vi "RS485_Data_Ctrl.vi"() -> ()   [LabVIEW 2016]
uses:
  <vilib>/Analysis/NI_AALBase.lvlib
  <vilib>/Instr/_visa.llb/VISA Set IO Buffer Mask.ctl
  <vilib>/Instr/_visa.llb/VISA Flush IO Buffer Mask.ctl
  <vilib>/ptbypt/NI_PtbyPt.lvlib
  GEN_2.lvlib
  GEN2_Stat_Addr.ctl
  GEN2_Config_Addr.ctl
  <vilib>/Analysis/1siggen.llb/Ramp Pattern by Samples.vi
  <vilib>/Analysis/3filter.llb/Filter Passband Type.ctl
  <vilib>/Analysis/3filter.llb/Zero Phase Filter (DBL).vi
  <vilib>/Instr/_visa.llb/VISA Configure Serial Port (Instr).vi
  <vilib>/Analysis/1siggen.llb/Ramp Pattern by Delta.vi
  <vilib>/event_ctls.llb/eventvkey.ctl
panel:
  out "Error":cluster{dbl, dbl, dbl[]}[](graph)=[{0.0, 0.005, array[4200 elements]}, {0.0, 0.005, array[4200 elements]}]
  out "Current (Iq)":cluster{dbl, dbl, dbl[]}[](graph)=[{0.0, 0.005, array[4200 elements]}, {0.0, 0.005, array[4200 elements]}]
  out "Iq":dbl=-0.4256019592285156
  in  "which_goal":bool[](array[boolean])=[FALSE, TRUE, TRUE, TRUE]
  in  "ESTOP":bool
  in  "Write Configs":bool
  out "Theta_dot":cluster{"Mean":dbl, "Std":dbl}={"Mean"=0.00022035774236428551, "Std"=0.024452840778427565} {"Std" format="%.4f"; "Mean" format="%.4f"}
  out "Theta_LP":cluster{"Mean":dbl, "Std":dbl}={"Mean"=-0.566546102927532, "Std"=2.22577060098394e-05} {"Std" format="%.4f"; "Mean" format="%.4f"}
  out "Id":cluster{"Mean":dbl, "Std":dbl}={"Mean"=-0.00010110904884186311, "Std"=0.00796473691732965} {"Std" format="%.4f"; "Mean" format="%.4f"}
  in  "MT":cluster{"Expected":sgl, "Tolerance":sgl}
  in  "Find MT":bool
  out "Errors":bool[](array[boolean])=[FALSE, FALSE, FALSE, FALSE, FALSE, FALSE, FALSE, TRUE]
  in  "All config":cluster{"Config Address":T1, dbl}[](array[cluster])=[{"Config Address"=0, 1.0}, {"Config Address"=1, 3.0}, {"Config Address"=2, 8000000.0}, {"Config Address"=3, -0.496978759765625}, {"Config Address"=4, 0.018400000408291817}, {"Config Address"=5, 0.006500000134110451}, {"Config Address"=6, 0.0}, {"Config Address"=7, 0.018400000408291817}, {"Config Address"=8, 0.006500000134110451}, {"Config Address"=9, 0.0}, {"Config Address"=10, 5.0}, {"Config Address"=11, 0.029999999329447746}, {"Config Address"=12, 0.0}, {"Config Address"=13, 10.0}, {"Config Address"=14, 0.0}, {"Config Address"=15, 0.0}, {"Config Address"=16, 100.0}, {"Config Address"=17, 0.0}, {"Config Address"=18, 1.0}, {"Config Address"=19, 5.0}, {"Config Address"=20, 10.0}, {"Config Address"=21, 10.0}, {"Config Address"=22, -3.0}, {"Config Address"=23, 3.0}, {"Config Address"=24, 6.0}, {"Config Address"=25, 60.0}, {"Config Address"=26, 0.0}, {"Config Address"=27, 80.0}, {"Config Address"=28, 100.0}] {"Config Address" items=["ID", "Mode", "Baudrate", "Homing Offset", "Id P gain", "Id I gain", "Id D gain", "Iq P gain", "Iq I gain", "Iq D gain", "Velo P gain", "Velo I gain", "Velo D gain", "Posi P gain", "Posi I gain", "Posi D gain", "DirectForce P", "DirectForce I", "DirectForce D", "Limit Acc Max", "Limit Iq Max", "Limit Velo Max", "Limit Posi Min", "Limit Posi Max", "Voltage Min", "Voltage Max", "Watchdog", "Temperature Low", "Temperature High"]}
  in  "SAVE":bool
  in  "Down_Key":bool
  in  "UP_Key":bool
  out "VKey":T2
  out "Vbus":dbl(graph)=11.93691349029541
  out "Error count":u64=1
  in  "Read Configs":bool
  out "Temperature":cluster{dbl, dbl, dbl}(graph)={27.25, 43.0078125, 41.5625}
  out "Iq":cluster{dbl, dbl}(graph)={-0.4256019592285156, -0.43746575713157654}
  out "Id":cluster{dbl, dbl}(graph)={0.0019982189405709505, 0.0}
  out "Theta":cluster{dbl, dbl}(graph)={-0.5665233731269836, -0.5707402229309082}
  out "Theta_dot":cluster{dbl, dbl}(graph)={-0.004696944262832403, 0.012627856805920601}
  in  "ID":u8=1
  in  "Read":bool=TRUE
  in  "PID0":bool
  in  "P0.001":bool
  in  "D0.5":bool
  in  "P0.0002":bool
  in  "send sine":bool
  in  "2state":bool
  in  "Chirp":i32(listbox)=3
  out "Waveform Graph":cluster{dbl, dbl, dbl[]}(graph)={0.0, 0.005, array[4200 elements]}
  in  "Sample_rate":dbl=200.0 format="%#_13g"
  out "Theta_LP":dbl=-0.5665233731269836
  in  "send chirp":bool
  in  "Enable":bool
  in  "DISABLE":bool
  in  "Write_Mode":bool
  in  "Mode":i32(listbox)=3
  in  "Write_Limits":bool
  in  "Limits":cluster{"Iq&Id":sgl, "Velo":sgl, "Acc":sgl}={"Iq&Id"=10.0, "Velo"=10.0, "Acc"=5.0}
  in  "Goal":T3
  in  "PID_F":cluster{"P":sgl, "I":sgl, "D":sgl}={"P"=100.0, "I"=0.0, "D"=1.0}
  in  "PID_P":cluster{"P":sgl, "I":sgl, "D":sgl}={"P"=10.0, "I"=0.0, "D"=0.0}
  out "Iq":cluster{"Mean":dbl, "Std":dbl}={"Mean"=-0.4106114786118269, "Std"=0.012899504647628292} {"Std" format="%.4f"; "Mean" format="%.4f"}
  in  "amplitude":dbl=2.0 format="%#_13g"
  in  "Time":dbl=20.0 format="%#_13g"
  in  "frq_2":dbl=0.2 format="%#_13g"
  in  "frq_1":dbl format="%#_13g"
  in  "stop":bool
  in  "Write_Goal":bool
  in  "PID_IqId":cluster{"P":sgl, "I":sgl, "D":sgl}={"P"=0.0184, "I"=0.0065, "D"=0.0}
  in  "PID_V":cluster{"P":sgl, "I":sgl, "D":sgl}={"P"=5.0, "I"=0.03, "D"=0.0}
  in  "Write_PID":bool
  in  "Baudrate":u32=8000000
  in  "Buffer Size":u32=150000
  in  "COM":refnum<visa-resource-name>="COM13"
  # "0: WARN COMM\n1: WARN OVTEMP\n2: ERR ABS POSI\n3: ERR WTCHDOG\n4: ERR JOINT LMT\n5: ERR HW FAULT\n6: ERR INIT"
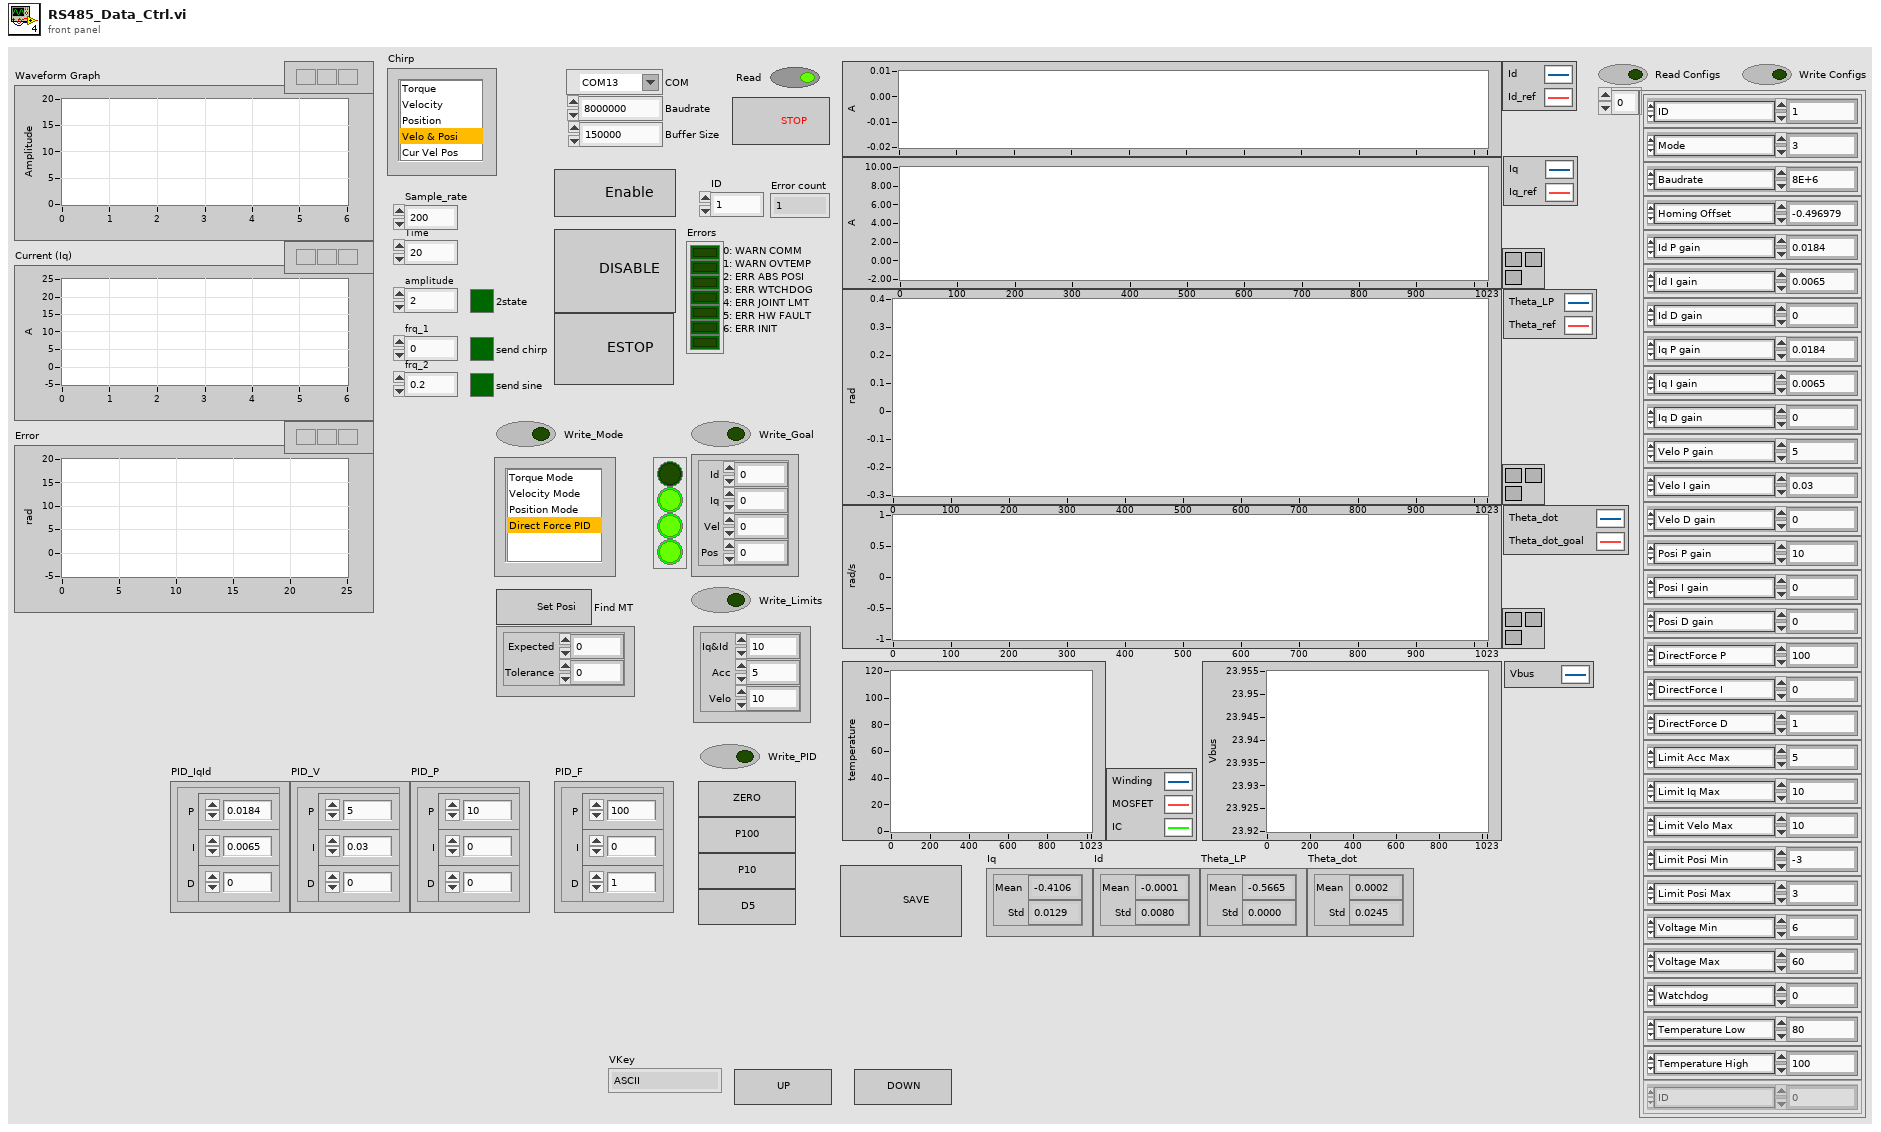
[diagram p1: front panel]
types:
  T1 = typedef "GEN_2.lvlib/GEN2_Config_Addr.ctl" = u8
  T2 = typedef "eventvkey.ctl" = enum16{"ASCII", "Enter", "Return", "Shift", "Ctrl", "Alt", "Cmd", "Opt", "Caps", "NumLock", "Clear", "Break", "Up", "Down", "Left", "Right", "Insert", "Delete", "Home", "End", "PageUp", "PageDown", "Escape", "Help", "Pause", "ScrollLock", "F1", "F2", "F3", "F4", "F5", "F6", "F7", "F8", "F9", "F10", "F11", "F12", "F13", "F14", "F15", "F16", "F17", "F18", "F19", "F20", "F21", "F22", "F23", "F24", "Play", "VolumeUp", "VolumeDown", "Mute", "Two Byte Char"}
  T3 = cluster{"Id":sgl, "Iq":sgl, "Pos":sgl, "Vel":sgl}
  T4 = typedef "NI_AALBase.lvlib/Filter Passband Type.ctl" = enum32{"Lowpass", "Highpass", "Bandpass", "Bandstop"}
  T5 = typedef "VISA Flush IO Buffer Mask.ctl" = u16
  T6 = typedef "VISA Set IO Buffer Mask.ctl" = u16
  T7 = typedef "GEN_2.lvlib/GEN2_Stat_Addr.ctl" = u8
  T8 = cluster{"filter structure":enum32{"IIR 2nd Order", "IIR 4th Order"}, "Reverse Coefficients":dbl[], "Forward Coefficients":dbl[]}
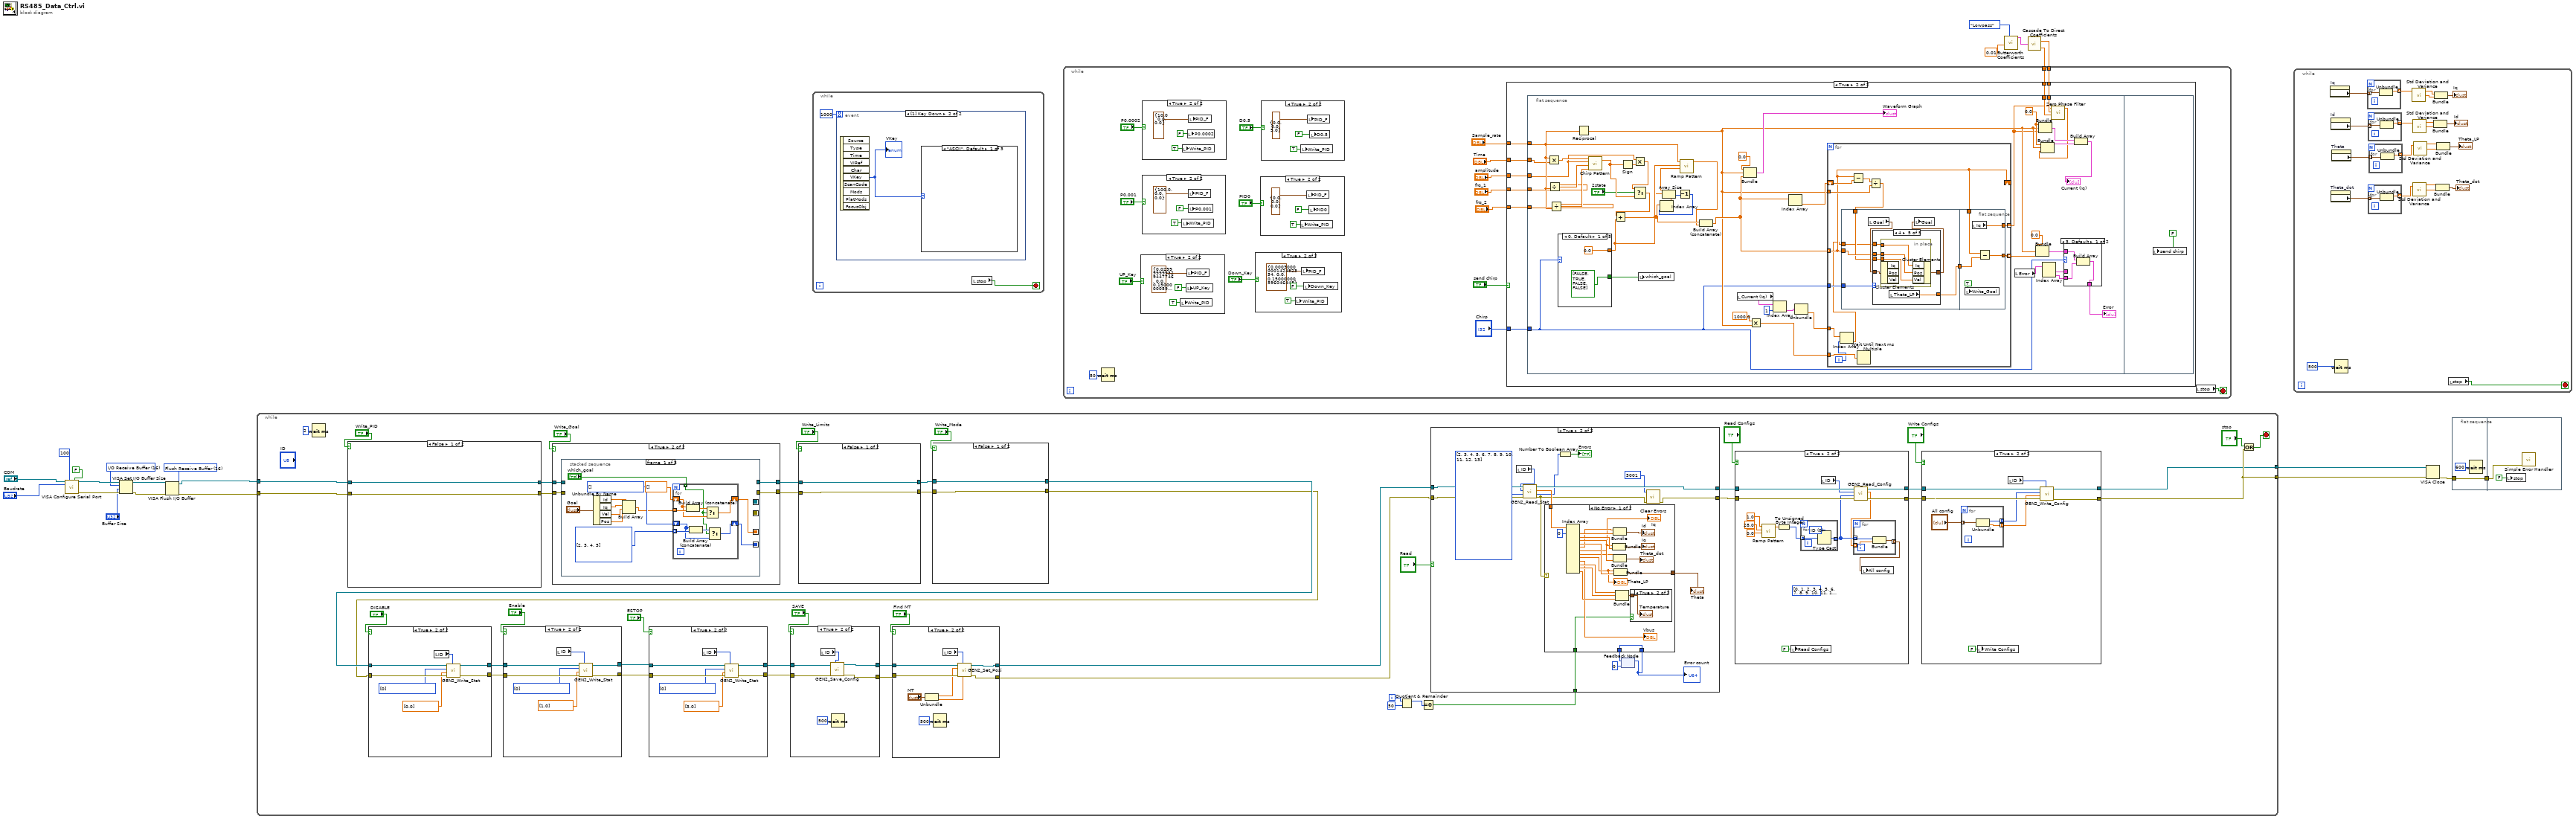
[diagram p0: block diagram]
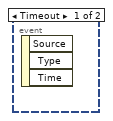
[diagram p2: hidden frame]
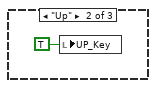
[diagram p3: hidden frame]
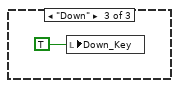
[diagram p4: hidden frame]
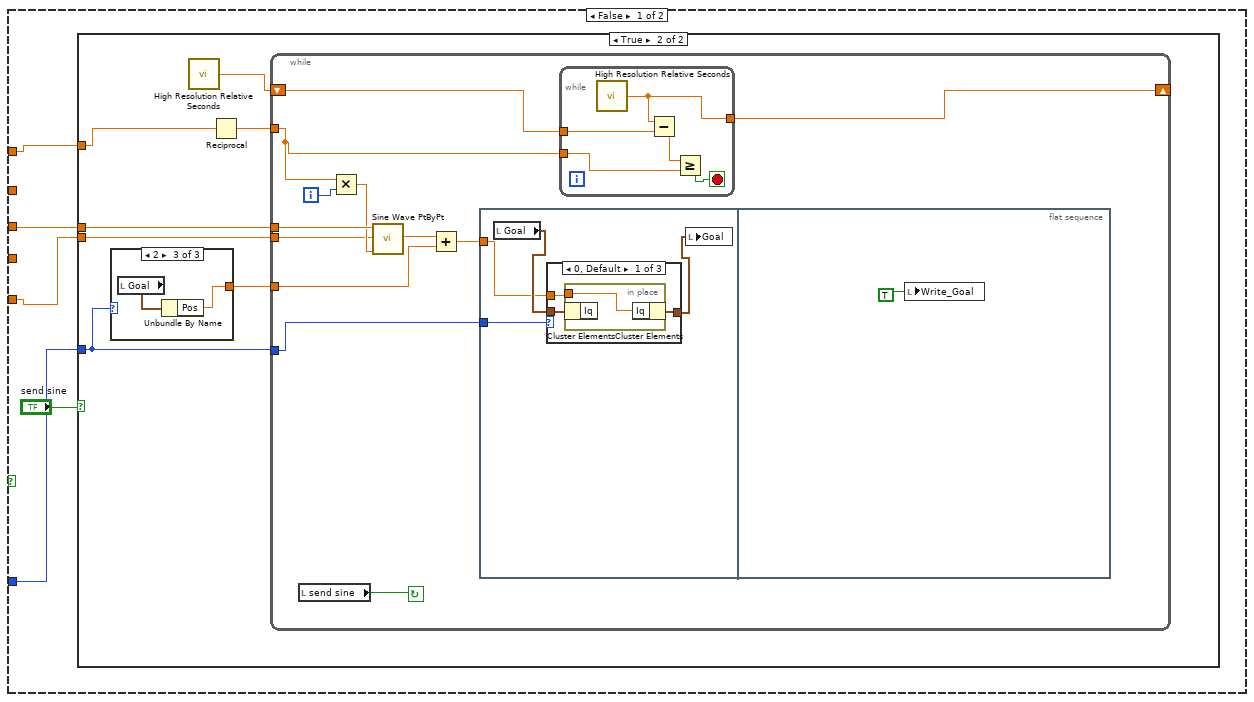
[diagram p11: hidden frame]
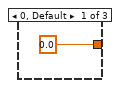
[diagram p13: hidden frame]
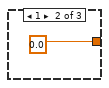
[diagram p14: hidden frame]
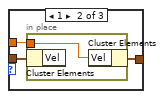
[diagram p15: hidden frame]
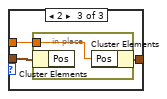
[diagram p16: hidden frame]
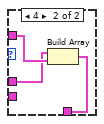
[diagram p17: hidden frame]
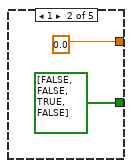
[diagram p18: hidden frame]
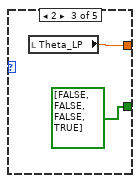
[diagram p19: hidden frame]
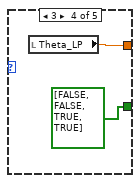
[diagram p20: hidden frame]
diagram:
  w8 = T5 16 items=["Flush Receive Buffer"=16, "Write Transmit Buffer to Device"=32, "Flush Receive Buffer (No I/O)"=64, "Flush Transmit Buffer"=128] ("Mask")
  w10 = T6 16 items=["I/O Receive Buffer"=16, "I/O Transmit Buffer"=32, "I/O Receive and Transmit Buffer"=48] ("Mask")
  n1 = call-poly "VISA Configure Serial Port"("VISA resource name"="COM", "timeout (10sec)"=u32 100, "Enable Termination\nChar (T)"=FALSE ("Enable Termination\nChar (T)"), "baud rate (9600)"="Baudrate") -> ("VISA resource name out"=w17:refnum<visa-resource-name>, "error out"=w16:errorcluster)  [unwired: 10 in]
  n2 = VISA Set I/O Buffer Size(VISA resource name=w17, mask (16)=w10, size (4096)="Buffer Size", error in (no error)=w16) -> (VISA resource name out=w6:refnum<visa-resource-name>, error out=w7:errorcluster)
  n3 = VISA Flush I/O Buffer(VISA resource name=w6, mask (16)=w8, error in (no error)=w7) -> (VISA resource name out=w11:refnum<visa-resource-name>, error out=w14:errorcluster)
  n4 = while {
    tunnel: w11 -> [w62]
    tunnel: w14 -> [w63]
    tunnel: [w31] -> w20
    tunnel: [w32] -> w19
    i -> [w36]
    stop <- w64 stop-if-true
    n5 = Wait (ms)(milliseconds to wait=u32 2) -> ()  [unwired: 1 out]
    n6 = case shown="False" "Write_PID" {
      tunnel: w62 -> [w254 w259]
      tunnel: w63 -> [w255 w258]
      tunnel: [w255 w257] -> w60
      tunnel: [w254 w256] -> w61
      frame False {
      }
      frame True {
        n7 = stacked-sequence {
          seq-local: [w270 _] -> [_ w291]
          seq-local: [w269 _] -> [_ w290]
          tunnel: w259 -> [w271 _]
          tunnel: w258 -> [w268 _]
          tunnel: [_ w290] -> w257
          tunnel: [_ w291] -> w256
          frame #0 {
            n8 = Cluster To Array(cluster="PID_IqId") -> (array=w263:sgl[])
            n9 = Cluster To Array(cluster="PID_V") -> (array=w262:sgl[])
            n10 = Cluster To Array(cluster="PID_P") -> (array=w261:sgl[])
            n11 = Cluster To Array(cluster="PID_F") -> (array=w260:sgl[])
            n12 = disable-structure shown="Enabled" {
              disable-tunnel: w271 -> [w282 w289]
              disable-tunnel: [w281 w288] -> w270
              disable-tunnel: [w279 w286] -> w269
              disable-tunnel: w268 -> [w278 w285]
              disable-tunnel: w263 -> [w276 _]
              disable-tunnel: w262 -> [w275 _]
              disable-tunnel: w261 -> [w274 _]
              disable-tunnel: w260 -> [w273 w283]
              frame Enabled {
                w277 = T1[] [4, 5, 6, 7, 8, 9, 10, 11, 12, 13, 14, 15, 16, 17, 18] items=["ID", "Mode", "Baudrate", "Homing Offset", "Id P gain", "Id I gain", "Id D gain", "Iq P gain", "Iq I gain", "Iq D gain", "Velo P gain", "Velo I gain", "Velo D gain", "Posi P gain", "Posi I gain", "Posi D gain", "DirectForce P", "DirectForce I", "DirectForce D", "Limit Id Max", "Limit Iq Max", "Limit Velo Max", "Limit Posi Min", "Limit Posi Max", "Voltage Min", "Voltage Max", "Watchdog", "Temperature Low", "Temperature High"] ("Config Addr")
                n13 = Build Array (concatenate)(w276, w276, w275, w274, w273) -> (w272:sgl[])
                n14 = local read "ID"() -> (w280:u8)
                n15 = call "GEN2_Write_Config.vi"("ID"=w280, "error in (no error)"=w278, "Data"=w272, "Config Addr"=w277, "VISA Refnum in"=w282) -> ("error out"=w279:errorcluster, "VISA Refnum out"=w281:refnum<visa-resource-name>)  [unwired: 5 in]
              }
              frame Disabled {
                w284 = T1[] [16, 17, 18] items=["ID", "Mode", "Baudrate", "Homing Offset", "Id P gain", "Id I gain", "Id D gain", "Iq P gain", "Iq I gain", "Iq D gain", "Velo P gain", "Velo I gain", "Velo D gain", "Posi P gain", "Posi I gain", "Posi D gain", "DirectForce P", "DirectForce I", "DirectForce D", "Limit Id Max", "Limit Iq Max", "Limit Velo Max", "Limit Posi Min", "Limit Posi Max", "Voltage Min", "Voltage Max", "Watchdog", "Temperature Low", "Temperature High"] ("Config Addr")
                n16 = local read "ID"() -> (w287:u8)
                n17 = call "GEN2_Write_Config.vi"("ID"=w287, "error in (no error)"=w285, "Data"=w283, "Config Addr"=w284, "VISA Refnum in"=w289) -> ("error out"=w286:errorcluster, "VISA Refnum out"=w288:refnum<visa-resource-name>)  [unwired: 5 in]
              }
            }
          }
          frame #1 {
            n18 = local write "Write_PID"(FALSE ("WriteP_PID")) -> ()
          }
        }
      }
    }
    n19 = case shown="True" "Write_Goal" {
      tunnel: w60 -> [w218 w222]
      tunnel: w61 -> [w217 w221]
      tunnel: [w218 w220] -> w57
      tunnel: [w217 w219] -> w58
      frame False {
      }
      frame True {
        n20 = stacked-sequence {
          seq-local: [_ w247 _] -> [_ _ w252]
          seq-local: [_ w246 _] -> [_ _ w251]
          seq-local: [w224 _ _] -> [_ w245 _]
          seq-local: [w223 _ _] -> [_ w244 _]
          tunnel: w222 -> [_ w249 _]
          tunnel: w221 -> [_ w248 _]
          tunnel: [_ _ w251] -> w220
          tunnel: [_ _ w252] -> w219
          frame #0 {
            w227 = T7[] [] items=["Torque Enable", "Homing Complete", "Goal Id", "Goal Iq", "Goal Velo", "Goal Posi", "Present Id", "Present Iq", "Present Velo", "Present Posi", "Bus Voltage", "Temperature Winding", "Temperature MOSFET", "Temperature IC", "Error Status"] ("Stat Addr")
            w225 = T7[] [2, 3, 4, 5] items=["Torque Enable", "Homing Complete", "Goal Id", "Goal Iq", "Goal Velo", "Goal Posi", "Present Id", "Present Iq", "Present Velo", "Present Posi", "Bus Voltage", "Temperature Winding", "Temperature MOSFET", "Temperature IC", "Error Status"] ("Stat Addr")
            n21 = Unbundle By Name("Goal") -> ("Id"=w229:sgl, "Iq"=w230:sgl, "Vel"=w231:sgl, "Pos"=w232:sgl)
            n22 = Build Array(w229, w230, w231, w232) -> (w226:sgl[])
            n23 = for {
              tunnel: "which_goal" -> [w236] mode=indexing
              shift-right: [w241] -> w224
              shift-left: sgl[] [] ("appended array") -> [w240]
              shift-right: [w235] -> w223
              shift-left: w227 -> [w237]
              tunnel: w226 -> [w243] mode=indexing
              tunnel: w225 -> [w238] mode=indexing
              n24 = Build Array (concatenate)(w240, w243) -> (w242:sgl[])
              n25 = Build Array (concatenate)(w237, w238) -> (w239:T7[])
              n26 = Select(t=w242, s=w236, f=w240) -> (s? t:f=w241:sgl[])
              n27 = Select(t=w239, s=w236, f=w237) -> (s? t:f=w235:T7[])
            }
          }
          frame #1 {
            n28 = local read "ID"() -> (w250:u8)
            n29 = call "GEN2_Write_Stat.vi"("ID"=w250, "error in (no error)"=w249, "Data"=w245, "Stat Addr"=w244, "VISA Refnum in"=w248) -> ("error out"=w246:errorcluster, "VISA Refnum out"=w247:refnum<visa-resource-name>)  [unwired: 5 in]
          }
          frame #2 {
            n30 = local write "Write_Goal"(FALSE ("WriteP_PID")) -> ()
          }
        }
      }
    }
    n31 = case shown="False" "Write_Limits" {
      tunnel: w57 -> [w161 w172]
      tunnel: w58 -> [w160 w171]
      tunnel: [w161 w164] -> w54
      tunnel: [w160 w165] -> w55
      frame False {
      }
      frame True {
        w162 = T1[] [20, 21, 19] items=["ID", "Mode", "Baudrate", "Homing Offset", "Id P gain", "Id I gain", "Id D gain", "Iq P gain", "Iq I gain", "Iq D gain", "Velo P gain", "Velo I gain", "Velo D gain", "Posi P gain", "Posi I gain", "Posi D gain", "DirectForce P", "DirectForce I", "DirectForce D", "Limit Acc Max", "Limit Iq Max", "Limit Velo Max", "Limit Posi Min", "Limit Posi Max", "Voltage Min", "Voltage Max", "Watchdog", "Temperature Low", "Temperature High"] ("Config Addr")
        n32 = Unbundle By Name("Limits") -> ("Iq&Id"=w166:sgl, "Velo"=w167:sgl, "Acc"=w163:sgl)
        n33 = Build Array(w166, w167, w163) -> (w168:sgl[])
        n34 = local read "ID"() -> (w169:u8)
        n35 = call "GEN2_Write_Config.vi"("ID"=w169, "error in (no error)"=w172, "Data"=w168, "Config Addr"=w162, "VISA Refnum in"=w171) -> ("error out"=w164:errorcluster, "VISA Refnum out"=w165:refnum<visa-resource-name>)  [unwired: 5 in]
      }
    }
    n36 = case shown="False" "Write_Mode" {
      tunnel: w54 -> [w151 w159]
      tunnel: w55 -> [w150 w158]
      tunnel: [w151 w152] -> w51
      tunnel: [w150 w153] -> w52
      frame False {
      }
      frame True {
        w156 = T1[] [1] items=["ID", "Mode", "Baudrate", "Homing Offset", "Id P gain", "Id I gain", "Id D gain", "Iq P gain", "Iq I gain", "Iq D gain", "Velo P gain", "Velo I gain", "Velo D gain", "Posi P gain", "Posi I gain", "Posi D gain", "DirectForce P", "DirectForce I", "DirectForce D", "Limit Id Max", "Limit Iq Max", "Limit Velo Max", "Limit Posi Min", "Limit Posi Max", "Voltage Min", "Voltage Max", "Watchdog", "Temperature Low", "Temperature High"] ("Config Addr")
        n37 = Build Array("Mode") -> (w155:i32[])
        n38 = local read "ID"() -> (w157:u8)
        n39 = call "GEN2_Write_Config.vi"("ID"=w157, "error in (no error)"=w159, "Data"=w155, "Config Addr"=w156, "VISA Refnum in"=w158) -> ("error out"=w152:errorcluster, "VISA Refnum out"=w153:refnum<visa-resource-name>)  [unwired: 5 in]
      }
    }
    n40 = case shown="True" "DISABLE" {
      tunnel: w51 -> [w142 w149]
      tunnel: w52 -> [w141 w148]
      tunnel: [w142 w143] -> w48
      tunnel: [w141 w144] -> w49
      frame False {
      }
      frame True {
        w147 = T7[] [0] items=["Torque Enable", "Homing Complete", "Goal Id", "Goal Iq", "Goal Velo", "Goal Posi", "Present Id", "Present Iq", "Present Velo", "Present Posi", "Bus Voltage", "Temperature Winding", "Temperature MOSFET", "Temperature IC", "Error Status"] ("Stat Addr")
        n41 = local read "ID"() -> (w145:u8)
        n42 = call "GEN2_Write_Stat.vi"("ID"=w145, "error in (no error)"=w149, "Data"=dbl[] [0.0], "Stat Addr"=w147, "VISA Refnum in"=w148) -> ("error out"=w143:errorcluster, "VISA Refnum out"=w144:refnum<visa-resource-name>)  [unwired: 5 in]
      }
    }
    n43 = case shown="True" "Enable" {
      tunnel: w48 -> [w133 w140]
      tunnel: w49 -> [w132 w139]
      tunnel: [w133 w134] -> w27
      tunnel: [w132 w135] -> w26
      frame False {
      }
      frame True {
        w136 = T7[] [0] items=["Torque Enable", "Homing Complete", "Goal Id", "Goal Iq", "Goal Velo", "Goal Posi", "Present Id", "Present Iq", "Present Velo", "Present Posi", "Bus Voltage", "Temperature Winding", "Temperature MOSFET", "Temperature IC", "Error Status"] ("Stat Addr")
        n44 = local read "ID"() -> (w138:u8)
        n45 = call "GEN2_Write_Stat.vi"("ID"=w138, "error in (no error)"=w140, "Data"=dbl[] [1.0], "Stat Addr"=w136, "VISA Refnum in"=w139) -> ("error out"=w134:errorcluster, "VISA Refnum out"=w135:refnum<visa-resource-name>)  [unwired: 5 in]
      }
    }
    n46 = case shown="True" "ESTOP" {
      tunnel: w27 -> [w69 w76]
      tunnel: w26 -> [w68 w75]
      tunnel: [w69 w70] -> w24
      tunnel: [w68 w71] -> w25
      frame False {
      }
      frame True {
        w72 = T7[] [0] items=["Torque Enable", "Homing Complete", "Goal Id", "Goal Iq", "Goal Velo", "Goal Posi", "Present Id", "Present Iq", "Present Velo", "Present Posi", "Bus Voltage", "Temperature Winding", "Temperature MOSFET", "Temperature IC", "Error Status"] ("Stat Addr")
        n47 = local read "ID"() -> (w74:u8)
        n48 = call "GEN2_Write_Stat.vi"("ID"=w74, "error in (no error)"=w76, "Data"=dbl[] [3.0], "Stat Addr"=w72, "VISA Refnum in"=w75) -> ("error out"=w70:errorcluster, "VISA Refnum out"=w71:refnum<visa-resource-name>)  [unwired: 5 in]
      }
    }
    n49 = case shown="True" "SAVE" {
      tunnel: w25 -> [w103 w109]
      tunnel: w24 -> [w102 w108]
      tunnel: [w103 w105] -> w41
      tunnel: [w102 w104] -> w40
      frame False {
      }
      frame True {
        n50 = local read "ID"() -> (w107:u8)
        n51 = call "GEN2_Save_Config.vi"("ID"=w107, "error in (no error)"=w108, "VISA Refnum in"=w109) -> ("error out"=w104:errorcluster, "VISA Refnum out"=w105:refnum<visa-resource-name>)  [unwired: 7 in]
        n52 = Wait (ms)(milliseconds to wait=u32 500) -> ()  [unwired: 1 out]
      }
    }
    n53 = case shown="True" "Find MT" {
      tunnel: w41 -> [w92 w101]
      tunnel: w40 -> [w91 w100]
      tunnel: [w92 w94] -> w39
      tunnel: [w91 w93] -> w38
      frame False {
      }
      frame True {
        n54 = Unbundle("MT") -> ("Expected"=w97:sgl, "Tolerance"=w96:sgl)
        n55 = Wait (ms)(milliseconds to wait=u32 500) -> ()  [unwired: 1 out]
        n56 = local read "ID"() -> (w95:u8)
        n57 = call "GEN2_Set_Posi.vi"("Tolerance"=w96, "ID"=w95, "error in (no error)"=w100, "Expected Theta"=w97, "VISA Refnum in"=w101) -> ("error out"=w93:errorcluster, "VISA Refnum out"=w94:refnum<visa-resource-name>)  [unwired: 5 in]
      }
    }
    n58 = Quotient & Remainder(x=w36, y=50) -> (x-y*floor(x/y)=w34:i32)  [unwired: 1 out]
    n59 = Equal To 0?(x=w34) -> (x = 0?=w33:bool)
    n60 = case shown="True" "Read" {
      tunnel: [w174 w185] -> w43
      tunnel: w38 -> [w173 w189]
      tunnel: w39 -> [w174 w190]
      tunnel: [w173 w182] -> w44
      tunnel: w33 -> [_ w175]
      frame False {
      }
      frame True {
        w187 = T7[] [2, 3, 4, 5, 6, 7, 8, 9, 10, 11, 12, 13] items=["Torque Enable", "Homing Complete", "Goal Id", "Goal Iq", "Goal Velo", "Goal Posi", "Present Id", "Present Iq", "Present Velo", "Present Posi", "Bus Voltage", "Temperature Winding", "Temperature MOSFET", "Temperature IC", "Error Status"] ("Stat Address")
        n61 = local read "ID"() -> (w188:u8)
        n62 = call "GEN2_Read_Stat.vi"("error in (no error)"=w189, "Stat Address"=w187, "ID"=w188, "VISA Refnum in"=w190) -> ("error out"=w183:errorcluster, "ERROR"=w177:u8, "Data"=w186:dbl[], "VISA Refnum out"=w185:refnum<visa-resource-name>)  [unwired: 4 in]
        n63 = Number To Boolean Array(number=w177) -> (Boolean array=→"Errors":bool[])
        n64 = feedback #1(u64 0) -> (w180:u64)
        n65 = case shown="No Error" w183 {
          tunnel: w186 -> [w207 _]
          tunnel: w180 -> [w193 w216]
          tunnel: [w193 w215] -> w179
          tunnel: [w192 w214] -> w178
          tunnel: w175 -> [w191 _]
          frame No Error {
            n66 = Index Array(array=w207, index #1=0 ("index")) -> (element #1=w206:dbl, element #2=w205:dbl, element #3=w204:dbl, element #4=w203:dbl, element #5=w202:dbl, element #6=w201:dbl, element #7=w200:dbl, element #8=w199:dbl, element #9=→"Vbus":dbl, element #10=w195:dbl, element #11=w196:dbl, element #12=w197:dbl)  [unwired: 11 in]
            "Theta_LP" <- w199
            "Iq" <- w201
            n67 = Bundle(w201, w205) -> (→"Iq":cluster{dbl, dbl})  [unwired: 1 in]
            n68 = Bundle(w200, w204) -> (→"Theta_dot":cluster{dbl, dbl})  [unwired: 1 in]
            n69 = Bundle(w202, w206) -> (→"Id":cluster{dbl, dbl})  [unwired: 1 in]
            n70 = Bundle(w199, w203) -> (w192:cluster{dbl, dbl})  [unwired: 1 in]
            n71 = Bundle(w195, w196, w197) -> (w198:cluster{dbl, dbl, dbl})  [unwired: 1 in]
            n72 = case shown="True" w191 {
              tunnel: w198 -> [_ w212]
              frame False {
              }
              frame True {
                "Temperature" <- w212
              }
            }
          }
          frame Error {
            w213 = nan
            n73 = Increment(x=w216) -> (x+1=w215:u64)
            n74 = Bundle(w213, w213) -> (w214:cluster{dbl, dbl})  [unwired: 1 in]
          }
        }
        "Error count" <- w179
        "Theta" <- w178
        n75 = feedback-in #1(w179) -> ()
        n76 = call <vilib>:"Clear Errors.vi"("error in (no error)"=w183, "specific error code to clear (0: all)"=5001) -> ("error out"=w182:errorcluster)  [unwired: 4 in, 1 out]
      }
    }
    n77 = case shown="True" "Read Configs" {
      tunnel: w44 -> [w110 w124]
      tunnel: w43 -> [w111 w123]
      tunnel: [w110 w121] -> w29
      tunnel: [w111 w120] -> w30
      frame False {
      }
      frame True {
        (unwired) T1[] [0, 1, 2, 3, 4, 5, 6, 7, 8, 9, 10, 11, 12, 13, 14, 15, 16, 17, 18, 19, 20, 21, 22, 23, 24, 25, 26, 27, 28] items=["ID", "Mode", "Baudrate", "Homing Offset", "Id P gain", "Id I gain", "Id D gain", "Iq P gain", "Iq I gain", "Iq D gain", "Velo P gain", "Velo I gain", "Velo D gain", "Posi P gain", "Posi I gain", "Posi D gain", "DirectForce P", "DirectForce I", "DirectForce D", "Limit Id Max", "Limit Iq Max", "Limit Velo Max", "Limit Posi Min", "Limit Posi Max", "Voltage Min", "Voltage Max", "Watchdog", "Temperature Low", "Temperature High"] ("Array")
        n78 = call-poly <vilib>:"Ramp Pattern.vi"("start"=0.0, "end"=28.0, "delta"=1.0) -> ("Ramp Pattern"=w116:dbl[])  [unwired: 6 in, 2 out]
        n79 = To Unsigned Byte Integer(number=w116) -> (unsigned 8bit integer=w115:u8[])
        n80 = local write "Read Configs"(FALSE ("Read Config")) -> ()
        n81 = for {
          tunnel: w115 -> [w131] mode=indexing
          tunnel: [w130] -> w114 mode=indexing
          w129 = T1 0 items=["ID", "Mode", "Baudrate", "Homing Offset", "Id P gain", "Id I gain", "Id D gain", "Iq P gain", "Iq I gain", "Iq D gain", "Velo P gain", "Velo I gain", "Velo D gain", "Posi P gain", "Posi I gain", "Posi D gain", "DirectForce P", "DirectForce I", "DirectForce D", "Limit Id Max", "Limit Iq Max", "Limit Velo Max", "Limit Posi Min", "Limit Posi Max", "Voltage Min", "Voltage Max", "Watchdog", "Temperature Low", "Temperature High"] ("Config Address")
          n82 = Type Cast(type=w129, x=w131) -> (*(type *) &x=w130:T1)
        }
        n83 = local read "ID"() -> (w122:u8)
        n84 = call "GEN2_Read_Config.vi"("error in (no error)"=w124, "Config Address"=w114, "ID"=w122, "VISA Refnum in"=w123) -> ("error out"=w121:errorcluster, "Data"=w113:dbl[], "VISA Refnum out"=w120:refnum<visa-resource-name>)  [unwired: 4 in, 1 out]
        n85 = for {
          tunnel: w114 -> [w128] mode=indexing
          tunnel: w113 -> [w127] mode=indexing
          tunnel: [w126] -> w112 mode=indexing
          n86 = Bundle("Config Address"=w128, w127) -> (w126:cluster{"Config Address":T1, dbl})  [unwired: 1 in]
        }
        n87 = local write "All config"(w112) -> ()
      }
    }
    n88 = case shown="True" "Write Configs" {
      tunnel: w29 -> [w77 w85]
      tunnel: w30 -> [w78 w86]
      tunnel: [w77 w83] -> w32
      tunnel: [w78 w84] -> w31
      frame False {
      }
      frame True {
        n89 = for {
          tunnel: "All config" -> [w90] mode=indexing
          tunnel: [w89] -> w80 mode=indexing
          tunnel: [w88] -> w79 mode=indexing
          n90 = Unbundle(w90) -> ("Config Address"=w89:T1, w88:dbl)
        }
        n91 = local write "Write Configs"(FALSE ("Read Config")) -> ()
        n92 = local read "ID"() -> (w82:u8)
        n93 = call "GEN2_Write_Config.vi"("ID"=w82, "error in (no error)"=w85, "Data"=w79, "Config Addr"=w80, "VISA Refnum in"=w86) -> ("error out"=w83:errorcluster, "VISA Refnum out"=w84:refnum<visa-resource-name>)  [unwired: 5 in]
      }
    }
    n94 = Or(x="stop", y=w32) -> (x .or. y?=w64:bool)
  }
  n95 = while {
    stop <- w294 stop-if-true
    n96 = event shown="[1] Key Down" {
      selector: _ -> [_ _]
      dyn-events: _ -> [_ _]
      timeout: 1000 -> [_ _]
      event Timeout {
        n97 = event-data() -> ()  [unwired: 1 in, 3 out]
      }
      event Key Down {
        n98 = event-data() -> ("VKey"=w295:T2)  [unwired: 1 in, 9 out]
        "VKey" <- w295
        n99 = case shown="\"ASCII\", Default" w295 {
          frame "ASCII", Default {
          }
          frame "Up" {
            n100 = local write "UP_Key"(TRUE ("P0.0002")) -> ()
          }
          frame "Down" {
            n101 = local write "Down_Key"(TRUE ("P0.0002")) -> ()
          }
        }
      }
    }
    n102 = local read "stop"() -> (w294:bool)
  }
  n103 = call <vilib>:"Butterworth Coefficients.vi"("filter type"=Filter_Passband_Type."Lowpass", "low cutoff freq: fl"=0.01) -> ("IIR Filter Cluster"=w4:T8)  [unwired: 8 in, 1 out]
  n104 = call <vilib>:"Cascade To Direct Coefficients.vi"("IIR Filter Cluster"=w4) -> ("Reverse Coefficients"=w1:dbl[], "Forward Coefficients"=w2:dbl[])
  n105 = while {
    tunnel: w2 -> [w299]
    tunnel: w1 -> [w298]
    stop <- w314 stop-if-true
    n106 = Wait (ms)(milliseconds to wait=u32 50) -> ()  [unwired: 1 out]
    n107 = case shown="True" "UP_Key" {
      frame False {
      }
      frame True {
        n108 = local write "Write_PID"(TRUE ("Write_PID")) -> ()
        n109 = local write "UP_Key"(FALSE ("P0.0002")) -> ()
        n110 = local write "PID_F"(cluster{"P":sgl, "I":sgl, "D":sgl} {"P"=0.03, "I"=0.0, "D"=0.15} ("PID_F 2")) -> ()
      }
    }
    n111 = case shown="True" "P0.001" {
      frame False {
      }
      frame True {
        n112 = local write "Write_PID"(TRUE ("Write_PID")) -> ()
        n113 = local write "PID_F"(cluster{"P":sgl, "I":sgl, "D":sgl} {"P"=100.0, "I"=0.0, "D"=0.0} ("PID_F 2")) -> ()
        n114 = local write "P0.001"(FALSE ("P0.0002")) -> ()
      }
    }
    n115 = case shown="True" "P0.0002" {
      frame False {
      }
      frame True {
        n116 = local write "Write_PID"(TRUE ("Write_PID")) -> ()
        n117 = local write "P0.0002"(FALSE ("P0.0002")) -> ()
        n118 = local write "PID_F"(cluster{"P":sgl, "I":sgl, "D":sgl} {"P"=10.0, "I"=0.0, "D"=0.0} ("PID_F 2")) -> ()
      }
    }
    n119 = case shown="True" "Down_Key" {
      frame False {
      }
      frame True {
        n120 = local write "Write_PID"(TRUE ("Write_PID")) -> ()
        n121 = local write "PID_F"(cluster{"P":sgl, "I":sgl, "D":sgl} {"P"=0.0003, "I"=0.0, "D"=0.15} ("PID_F 2")) -> ()
        n122 = local write "Down_Key"(FALSE ("P0.0002")) -> ()
      }
    }
    n123 = case shown="True" "PID0" {
      frame False {
      }
      frame True {
        n124 = local write "Write_PID"(TRUE ("Write_PID")) -> ()
        n125 = local write "PID_F"(cluster{"P":sgl, "I":sgl, "D":sgl} {"P"=0.0, "I"=0.0, "D"=0.0} ("PID_F 2")) -> ()
        n126 = local write "PID0"(FALSE ("P0.0002")) -> ()
      }
    }
    n127 = case shown="True" "D0.5" {
      frame False {
      }
      frame True {
        n128 = local write "Write_PID"(TRUE ("Write_PID")) -> ()
        n129 = local write "PID_F"(cluster{"P":sgl, "I":sgl, "D":sgl} {"P"=0.0, "I"=0.0, "D"=5.0} ("PID_F 2")) -> ()
        n130 = local write "D0.5"(FALSE ("P0.0002")) -> ()
      }
    }
    n131 = case shown="True" "send chirp" {
      tunnel: "Chirp" -> [w334 w390]
      tunnel: "Sample_rate" -> [w336 w389]
      tunnel: "Time" -> [_ w388]
      tunnel: "amplitude" -> [w335 w387]
      tunnel: "frq_1" -> [_ w386]
      tunnel: "frq_2" -> [w333 w385]
      tunnel: w299 -> [_ w384]
      tunnel: w298 -> [_ w383]
      frame False {
        n132 = case shown="True" "send sine" {
          tunnel: w336 -> [_ w340]
          tunnel: w335 -> [_ w341]
          tunnel: w334 -> [_ w343]
          tunnel: w333 -> [_ w344]
          frame False {
          }
          frame True {
            n133 = case shown="2" w343 {
              tunnel: [0.0 ("x") 0.0 ("x") w347] -> w342
              frame 0, Default {
              }
              frame 1 {
              }
              frame 2 {
                n134 = local read "Goal"() -> (w348:T3)
                n135 = Unbundle By Name(w348) -> ("Pos"=w347:sgl)
              }
            }
            n136 = call <vilib>:"High Resolution Relative Seconds.vi"() -> ("relative seconds"=w338:dbl)
            n137 = Reciprocal(x=w340) -> (1/x=w339:dbl)
            n138 = while {
              tunnel: w341 -> [w360]
              tunnel: w343 -> [w353]
              tunnel: w344 -> [w357]
              tunnel: w342 -> [w352]
              tunnel: w339 -> [w349]
              shift-right: [w351] -> _
              shift-left: w338 -> [w350]
              i -> [w359]
              stop <- w356 continue-if-true
              n139 = local read "send sine"() -> (w356:bool)
              n140 = Multiply(x=w349, y=w359) -> (x*y=w358:dbl)
              n141 = call <vilib>:"Sine Wave PtByPt.vi"("time"=w358, "frequency"=w357, "amplitude"=w360) -> ("sine wave"=w355:dbl)  [unwired: 1 in]
              n142 = Add(x=w355, y=w352) -> (x+y=w354:dbl)
              n143 = flat-sequence {
                tunnel: w354 -> [w368]
                tunnel: w353 -> [w367]
                frame #0 {
                  n144 = local read "Goal"() -> (w369:T3)
                  n145 = case shown="0, Default" w367 {
                    tunnel: w369 -> [w372 w376 w380]
                    tunnel: w368 -> [w370 w374 w379]
                    tunnel: [w371 w375 w378] -> w366
                    frame 0, Default {
                      n146 = in-place {
                        in-place-border: w370 -> [w373]
                        n147 = in-place-cluster #2(w372) -> ()  [unwired: 1 out]
                        n148 = in-place-cluster #2("Iq"=w373) -> (w371:T3)
                      }
                    }
                    frame 1 {
                      n149 = in-place {
                        in-place-border: w374 -> [w377]
                        n150 = in-place-cluster #3(w376) -> ()  [unwired: 1 out]
                        n151 = in-place-cluster #3("Vel"=w377) -> (w375:T3)
                      }
                    }
                    frame 2 {
                      n152 = in-place {
                        in-place-border: w379 -> [w381]
                        n153 = in-place-cluster #4(w380) -> ()  [unwired: 1 out]
                        n154 = in-place-cluster #4("Pos"=w381) -> (w378:T3)
                      }
                    }
                  }
                  n155 = local write "Goal"(w366) -> ()
                }
                frame #1 {
                  n156 = local write "Write_Goal"(TRUE ("Write_Dst")) -> ()
                }
              }
              n157 = while {
                tunnel: [w365] -> w351
                tunnel: w350 -> [w364]
                tunnel: w349 -> [w361]
                stop <- w362 stop-if-true
                n158 = call <vilib>:"High Resolution Relative Seconds.vi"() -> ("relative seconds"=w365:dbl)
                n159 = Subtract(x=w365, y=w364) -> (x-y=w363:dbl)
                n160 = Greater Or Equal?(x=w363, y=w361) -> (x >= y?=w362:bool)
              }
            }
          }
        }
      }
      frame True {
        n161 = flat-sequence {
          tunnel: w390 -> [w395]
          tunnel: w389 -> [w419]
          tunnel: w388 -> [w418]
          tunnel: w387 -> [w417]
          tunnel: w386 -> [w416]
          tunnel: w385 -> [w415]
          tunnel: w384 -> [w400]
          tunnel: w383 -> [w399]
          frame #0 {
            w402 = 0.0
            n162 = Multiply(x=w419, y=w418) -> (x*y=w434:dbl)
            n163 = Divide(x=w416, y=w419) -> (x/y=w436:dbl)
            n164 = Divide(x=w415, y=w419) -> (x/y=w435:dbl)
            n165 = case shown="0, Default" w395 {
              tunnel: [0.0 ("x") 0.0 ("x") w449 w451 w453] -> w423
              tunnel: [bool[] [FALSE, TRUE, FALSE, FALSE] ("which_goal") bool[] [FALSE, FALSE, TRUE, FALSE] ("which_goal") bool[] [FALSE, FALSE, FALSE, TRUE] ("which_goal") bool[] [FALSE, FALSE, TRUE, TRUE] ("which_goal") bool[] [FALSE, TRUE, TRUE, TRUE] ("which_goal")] -> w414
              frame 0, Default {
              }
              frame 1 {
              }
              frame 2 {
                n166 = local read "Theta_LP"() -> (w449:dbl)
              }
              frame 3 {
                n167 = local read "Theta_LP"() -> (w451:dbl)
              }
              frame 4 {
                n168 = local read "Theta_LP"() -> (w453:dbl)
              }
            }
            n169 = Reciprocal(x=w419) -> (1/x=w401:dbl)
            n170 = call <vilib>:"Chirp Pattern.vi"("f2"=w435, "f1"=w436, "amplitude"=w417, "samples"=w434) -> ("Chirp Pattern"=w428:dbl[])  [unwired: 1 out]
            n171 = Sign(1:w428) -> (0:w430:dbl[])
            n172 = Multiply(x=w417, y=w430) -> (x*y=w429:dbl[])
            n173 = Select(t=w429, s="2state", f=w428) -> (s? t:f=w427:dbl[])
            n174 = Add(x=w427, y=w423) -> (x+y=w421:dbl[])
            n175 = local write "which_goal"(w414) -> ()
            n176 = Array Size(array=w421) -> (size(s)=w425:i32)
            n177 = Decrement(x=w425) -> (x-1=w424:i32)
            n178 = Index Array(array=w421, index=w424) -> (element=w422:dbl)
            n179 = call-poly <vilib>:"Ramp Pattern.vi"("start"=w422, "end"=w423, "samples"=w419) -> ("Ramp Pattern"=w420:dbl[])  [unwired: 7 in, 1 out]
            n180 = Build Array (concatenate)(w421, w420) -> (w413:dbl[])
            n181 = local read "Current (Iq)"() -> (w406:cluster{dbl, dbl, dbl[]}[])
            n182 = Bundle(0.0, w401, w413) -> (→"Waveform Graph":cluster{dbl, dbl, dbl[]})  [unwired: 1 in]
            n183 = Multiply(x=1000.0, y=w401) -> (x*y=w432:dbl)
            n184 = Index Array(array=w406, index=1) -> (element=w404:cluster{dbl, dbl, dbl[]})
            n185 = Index Array(array=w413) -> (element=w412:dbl)  [unwired: 1 in]
            n186 = Unbundle(w404) -> (w409:dbl[])  [unwired: 2 out]
            n187 = for {
              tunnel: w413 -> [w458] mode=indexing
              tunnel: w432 -> [w466]
              tunnel: w395 -> [w465]
              shift-right: [w458] -> _
              shift-left: w412 -> [w464]
              tunnel: w401 -> [w462]
              tunnel: [w460] -> w398 mode=indexing
              tunnel: [w457] -> w410 mode=indexing
              tunnel: w409 -> [w456]
              i -> [w455]
              n188 = Index Array(array=w456, index=w455) -> (element=w454:dbl)
              n189 = flat-sequence {
                tunnel: w458 -> [w472]
                tunnel: w465 -> [w471]
                tunnel: w461 -> [w469]
                tunnel: [w468] -> w459
                tunnel: w454 -> [w467]
                tunnel: [w506] -> w460
                tunnel: w459 -> [w505]
                tunnel: w458 -> [w504]
                tunnel: [w503] -> w457
                frame #0 {
                  n190 = local read "Goal"() -> (w473:T3)
                  n191 = case shown="4" w471 {
                    tunnel: w473 -> [w476 w480 w485 w491 w499]
                    tunnel: w472 -> [w474 w478 w484 w490 w498]
                    tunnel: [w475 w479 w483 w489 w497] -> w470
                    tunnel: w469 -> [_ _ _ w488 w496]
                    tunnel: [_ _ w482 w487 w495] -> w468
                    tunnel: w467 -> [_ _ _ _ w494]
                    frame 0, Default {
                      n192 = in-place {
                        in-place-border: w474 -> [w477]
                        n193 = in-place-cluster #5(w476) -> ()  [unwired: 1 out]
                        n194 = in-place-cluster #5("Iq"=w477) -> (w475:T3)
                      }
                    }
                    frame 1 {
                      n195 = in-place {
                        in-place-border: w478 -> [w481]
                        n196 = in-place-cluster #6(w480) -> ()  [unwired: 1 out]
                        n197 = in-place-cluster #6("Vel"=w481) -> (w479:T3)
                      }
                    }
                    frame 2 {
                      n198 = in-place {
                        in-place-border: w484 -> [w486]
                        n199 = in-place-cluster #7(w485) -> ()  [unwired: 1 out]
                        n200 = in-place-cluster #7("Pos"=w486) -> (w483:T3)
                      }
                      n201 = local read "Theta_LP"() -> (w482:dbl)
                    }
                    frame 3 {
                      n202 = in-place {
                        in-place-border: w490 -> [w493]
                        in-place-border: w488 -> [w492]
                        n203 = in-place-cluster #8(w491) -> ()  [unwired: 2 out]
                        n204 = in-place-cluster #8("Pos"=w493, "Vel"=w492) -> (w489:T3)
                      }
                      n205 = local read "Theta_LP"() -> (w487:dbl)
                    }
                    frame 4 {
                      n206 = in-place {
                        in-place-border: w498 -> [w502]
                        in-place-border: w496 -> [w501]
                        in-place-border: w494 -> [w500]
                        n207 = in-place-cluster #9(w499) -> ()  [unwired: 3 out]
                        n208 = in-place-cluster #9("Iq"=w500, "Pos"=w502, "Vel"=w501) -> (w497:T3)
                      }
                      n209 = local read "Theta_LP"() -> (w495:dbl)
                    }
                  }
                  n210 = local write "Goal"(w470) -> ()
                }
                frame #1 {
                  n211 = local write "Write_Goal"(TRUE ("Write_Dst")) -> ()
                  n212 = local read "Iq"() -> (w506:dbl)
                  n213 = Subtract(x=w504, y=w505) -> (x-y=w503:dbl)
                }
              }
              n214 = Subtract(x=w458, y=w464) -> (x-y=w463:dbl)
              n215 = Wait Until Next ms Multiple(millisecond multiple=w466) -> ()  [unwired: 1 out]
              n216 = Divide(x=w463, y=w462) -> (x/y=w461:dbl)
            }
            n217 = local read "Error"() -> (w396:cluster{dbl, dbl, dbl[]}[])
            n218 = Bundle(0.0, w401, w410) -> (w394:cluster{dbl, dbl, dbl[]})  [unwired: 1 in]
            n219 = Bundle(w402, w401, w398) -> (w408:cluster{dbl, dbl, dbl[]})  [unwired: 1 in]
            n220 = Index Array(array=w396) -> (element #1=w392:cluster{dbl, dbl, dbl[]}, element #2=w391:cluster{dbl, dbl, dbl[]})  [unwired: 2 in]
            n221 = call-poly <vilib>:"Zero Phase Filter.vi"("Forward Coefficients"=w400, "Reverse Coefficients"=w399, "X"=w398) -> ("Filtered X"=w397:dbl[])  [unwired: 7 in, 1 out]
            n222 = Bundle(w402, w401, "Filtered X"=w397) -> (w403:cluster{dbl, dbl, "Filtered X":dbl[]})  [unwired: 1 in]
            n223 = case shown="3, Default" w395 {
              tunnel: w394 -> [w440 w442]
              tunnel: [w438 w443] -> w393
              tunnel: w392 -> [_ w441]
              tunnel: w391 -> [w439 _]
              frame 3, Default {
                n224 = Build Array(w440, w439) -> (w438:cluster{dbl, dbl, dbl[]}[])
              }
              frame 4 {
                n225 = Build Array(w441, w442) -> (w443:cluster{dbl, dbl, dbl[]}[])
              }
            }
            "Error" <- w393
            n226 = Build Array(w408, w403) -> (→"Current (Iq)":cluster{dbl, dbl, "Filtered X":dbl[]}[])
          }
          frame #1 {
            n227 = local write "send chirp"(FALSE ("send chirp")) -> ()
          }
        }
      }
    }
    n228 = local read "stop"() -> (w314:bool)
  }
  n229 = while {
    stop <- w518 stop-if-true
    n230 = property on="Iq" class="WFChart (strict)"() -> ("History Data"=w530:cluster{dbl, dbl}[])  [unwired: 2 in, 2 out]
    n231 = property on="Id" class="WFChart (strict)"() -> ("History Data"=w529:cluster{dbl, dbl}[])  [unwired: 2 in, 2 out]
    n232 = property on="Theta_dot" class="WFChart (strict)"() -> ("History Data"=w515:cluster{dbl, dbl}[])  [unwired: 2 in, 2 out]
    n233 = property on="Theta" class="WFChart (strict)"() -> ("History Data"=w516:cluster{dbl, dbl}[])  [unwired: 2 in, 2 out]
    n234 = Wait (ms)(milliseconds to wait=u32 500) -> ()  [unwired: 1 out]
    n235 = for {
      tunnel: w530 -> [w538] mode=indexing
      tunnel: [w537] -> w528 mode=indexing
      n236 = Unbundle(w538) -> (w537:dbl)  [unwired: 1 out]
    }
    n237 = for {
      tunnel: w529 -> [w536] mode=indexing
      tunnel: [w535] -> w526 mode=indexing
      n238 = Unbundle(w536) -> (w535:dbl)  [unwired: 1 out]
    }
    n239 = for {
      tunnel: w515 -> [w531] mode=indexing
      tunnel: [w532] -> w512 mode=indexing
      n240 = Unbundle(w531) -> (w532:dbl)  [unwired: 1 out]
    }
    n241 = for {
      tunnel: w516 -> [w533] mode=indexing
      tunnel: [w534] -> w527 mode=indexing
      n242 = Unbundle(w533) -> (w534:dbl)  [unwired: 1 out]
    }
    n243 = call <vilib>:"Std Deviation and Variance.vi"("X"=w528) -> ("mean"=w525:dbl, "standard deviation"=w524:dbl)  [unwired: 1 in, 1 out]
    n244 = call <vilib>:"Std Deviation and Variance.vi"("X"=w526) -> ("mean"=w521:dbl, "standard deviation"=w520:dbl)  [unwired: 1 in, 1 out]
    n245 = call <vilib>:"Std Deviation and Variance.vi"("X"=w512) -> ("mean"=w514:dbl, "standard deviation"=w513:dbl)  [unwired: 1 in, 1 out]
    n246 = call <vilib>:"Std Deviation and Variance.vi"("X"=w527) -> ("mean"=w522:dbl, "standard deviation"=w523:dbl)  [unwired: 1 in, 1 out]
    n247 = Bundle("mean"=w521, "standard deviation"=w520) -> (→"Id":cluster{"mean":dbl, "standard deviation":dbl})  [unwired: 1 in]
    n248 = Bundle("mean"=w525, "standard deviation"=w524) -> (→"Iq":cluster{"mean":dbl, "standard deviation":dbl})  [unwired: 1 in]
    n249 = Bundle("mean"=w514, "standard deviation"=w513) -> (→"Theta_dot":cluster{"mean":dbl, "standard deviation":dbl})  [unwired: 1 in]
    n250 = Bundle("mean"=w522, "standard deviation"=w523) -> (→"Theta_LP":cluster{"mean":dbl, "standard deviation":dbl})  [unwired: 1 in]
    n251 = local read "stop"() -> (w518:bool)
  }
  n252 = VISA Close(VISA resource name=w20, error in (no error)=w19) -> (error out=w13:errorcluster)
  n253 = flat-sequence {
    tunnel: w13 -> [w540]
    tunnel: [w540] -> w12
    tunnel: w12 -> [w541]
    frame #0 {
      n254 = Wait (ms)(milliseconds to wait=u32 600) -> ()  [unwired: 1 out]
    }
    frame #1 {
      n255 = local write "stop"(FALSE ("stop")) -> ()
      n256 = call <vilib>:"Simple Error Handler.vi"("error in (no error)"=w541) -> ()  [unwired: 4 in, 5 out]
    }
  }
